vi "Scan Control View.vi"(0 "Model in":refnum<class "Model.lvclass">) -> ()   [LabVIEW 2016, in "M1M3SupportEUI_Views.lvlib"]
uses:
  M1M3SupportEUI_Views.lvlib
  Model/Model.lvclass
  M1M3 Support Events/M1M3 Support Events.lvclass/M1M3 Support Events.ctl
  SALLV_m1m3/DataTypes/logevent_DetailedState.ctl
  M1M3 Support Events/M1M3 Support Events.lvclass
  SALLV_m1m3/SALLV_m1m3.lvlib
panel:
  in  "DetailedState":T1(ring)
  in  "Send State":bool
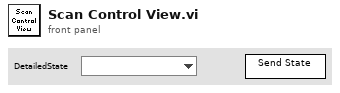
[diagram p1: front panel]
types:
  T1 = enum16{"", "DetailedState_DetailedStates_DisabledState", "DetailedState_DetailedStates_EnabledState", "DetailedState_DetailedStates_FaultState", "DetailedState_DetailedStates_OfflineState", "DetailedState_DetailedStates_StandbyState", "DetailedState_DetailedStates_ParkedState", "DetailedState_DetailedStates_RaisingState", "DetailedState_DetailedStates_ActiveState", "DetailedState_DetailedStates_LoweringState", "DetailedState_DetailedStates_EngineeringState", "DetailedState_DetailedStates_ParkedEngineeringState", "DetailedState_DetailedStates_RaisingEngineeringState", "DetailedState_DetailedStates_ActiveEngineeringState", "DetailedState_DetailedStates_LoweringEngineeringState", "DetailedState_DetailedStates_LoweringFaultState", "DetailedState_DetailedStates_ProfileHardpointCorrectionState"}
  T2 = typedef "M1M3SupportEUI_TypeDefs.lvlib/M1M3 Support Events.ctl" = cluster{"Inclinometer  Data":refnum<user-event>, "IMS Data":refnum<user-event>, "FA Status":refnum<user-event>, "SAL Connected":refnum<user-event>, "Accelerometer Data":refnum<user-event>, "OuterLoop Data":refnum<user-event>, "ErrorCode Event":refnum<user-event>, "InterlockStatus Event":refnum<user-event>, "InterlockWarning Event":refnum<user-event>, "Gyro Data":refnum<user-event>, "HP Actuator Info Event":refnum<user-event>, " FA Info Event":refnum<user-event>, "HP Monitor Info Event":refnum<user-event>, "FA Data":refnum<user-event>, "HP Actuator data":refnum<user-event>, "HP Monitor data":refnum<user-event>, "Air Supply Status Event":refnum<user-event>, "Air Supply Warning Event":refnum<user-event>, "Power Data":refnum<user-event>, "PID Data":refnum<user-event>, "PID Info Event":refnum<user-event>, "Power Status Event":refnum<user-event>, "Power Supply Status Event":refnum<user-event>, "Power Warning Event":refnum<user-event>, "Summary State Event":refnum<user-event>, "Detailed State Event":refnum<user-event>}
  T3 = typedef "SALLV_m1m3.lvlib/logevent_DetailedState.ctl" = cluster{"Timestamp":dbl, "DetailedState":enum16{"", "DetailedState_DetailedStates_DisabledState", "DetailedState_DetailedStates_EnabledState", "DetailedState_DetailedStates_FaultState", "DetailedState_DetailedStates_OfflineState", "DetailedState_DetailedStates_StandbyState", "DetailedState_DetailedStates_ParkedState", "DetailedState_DetailedStates_RaisingState", "DetailedState_DetailedStates_ActiveState", "DetailedState_DetailedStates_LoweringState", "DetailedState_DetailedStates_EngineeringState", "DetailedState_DetailedStates_ParkedEngineeringState", "DetailedState_DetailedStates_RaisingEngineeringState", "DetailedState_DetailedStates_ActiveEngineeringState", "DetailedState_DetailedStates_LoweringEngineeringState", "DetailedState_DetailedStates_LoweringFaultState", "DetailedState_DetailedStates_ProfileHardpointCorrectionState"}, "priority":i32}
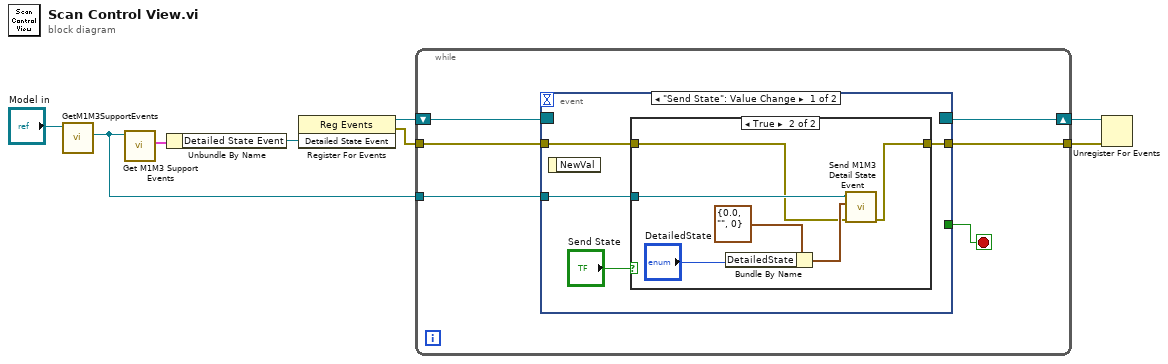
[diagram p0: block diagram]
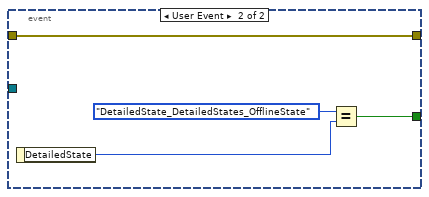
[diagram p3: hidden frame]
diagram:
  n1 = call "GetM1M3SupportEvents.vi"("Model in"="Model in") -> ("M1M3 Support Events out"=w2:refnum<class "M1M3 Support Events.lvclass">)  [unwired: 8 in, 2 out]
  n2 = call "Get M1M3 Support Events.vi"("M1M3 Support Events in"=w2) -> ("M1M3 Support Events"=w5:T2)  [unwired: 9 in, 1 out]
  n3 = Unbundle By Name(w5) -> ("Detailed State Event"=w4:refnum<user-event>)
  n4 = register-events(w4) -> (reference out=w8:refnum<event-registration>, error out=w1:errorcluster)  [unwired: 2 in]
  n5 = while {
    tunnel: [w9] -> w7
    tunnel: w2 -> [w14]
    shift-right: [w12] -> w6
    shift-left: w8 -> [w13]
    tunnel: w1 -> [w10]
    stop <- w11 stop-if-true
    n6 = event shown="[0] \"Send State\": Value Change" {
      selector: w13 -> [_ _]
      dyn-events: [_ _] -> w12
      timeout: _ -> [_ _]
      tunnel: w14 -> [w18 _]
      tunnel: [_ w29] -> w11
      tunnel: w10 -> [w16 w28]
      tunnel: [w15 w28] -> w9
      event "Send State": Value Change {
        n7 = event-data() -> ()  [unwired: 1 in, 1 out]
        n8 = case shown="True" "Send State" {
          tunnel: w18 -> [_ w23]
          tunnel: w16 -> [w19 w21]
          tunnel: [w19 w20] -> w15
          frame False {
          }
          frame True {
            n9 = Bundle By Name(cluster=T3 {"Timestamp"=0.0, "DetailedState"=enum."", "priority"=0} ("logevent_DetailedState"), "DetailedState"="DetailedState") -> (w22:T3)
            n10 = call "Send M1M3 Detail State Event.vi"("error in (no error)"=w21, "logevent_DetailedState"=w22, "M1M3 Support Events in"=w23) -> ("error out"=w20:errorcluster)  [unwired: 7 in, 1 out]
          }
        }
      }
      event User Event {
        n11 = event-data() -> ("DetailedState"=w27:T1)  [unwired: 1 in]
        n12 = Equal?(x=T1."DetailedState_DetailedStates_OfflineState", y=w27) -> (x = y?=w29:bool)
      }
    }
  }
  n13 = Unregister For Events(event registration refnum=w6, error in=w7) -> ()  [unwired: 1 out]
